vi "Bundle.vi"(8 "error in (no error)":errorcluster, 10 "Message":refnum<class "Message.lvclass">, 11 "Publish Msg in":refnum<class "Publish Msg.lvclass">) -> (0 "error out":errorcluster, 3 "Publish Msg out":refnum<class "Publish Msg.lvclass">)   [LabVIEW 2020, in "Publisher.lvlib" / "Publish Msg.lvclass"]
doc: "Populate the Publish Msg class."
uses:
  Publish Msg.lvclass
  PPL/HDH.Actor Framework.Core.Actor.lvlibp/1abvi3w/vi.lib/ActorFramework/Message/Message.lvclass
  Publish Msg.lvclass/Publish Msg.ctl
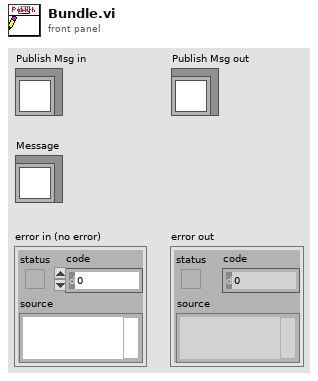
[diagram p1: front panel]
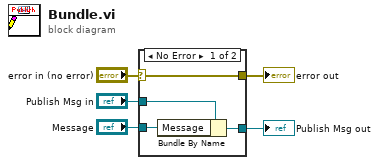
[diagram p0: block diagram]
diagram:
  n1 = case shown="No Error" "error in (no error)" {
    selector: "error in (no error)" -> [w9 w10]
    tunnel: [w9 w10] -> w4
    tunnel: [w7 w11] -> w2
    tunnel: "Publish Msg in" -> [w8 w11]
    tunnel: "Message" -> [w6 _]
    frame No Error {
      n2 = Bundle By Name(cluster=w8, "Message"=w6) -> (w7:refnum<class "Publish Msg.lvclass">)
    }
    frame Error {
    }
  }
  "error out" <- w4
  "Publish Msg out" <- w2
